vi "Test Passing Method.vi"(8 "error in (no error)":errorcluster, 11 "Test In Library in":refnum<class "Test In Library.lvclass">) -> (0 "error out":errorcluster, 3 "Test In Library out":refnum<class "Test In Library.lvclass">)   [LabVIEW 2020, in "library.lvlib" / "Test In Library.lvclass"]
uses:
  Test In Library.lvclass
  Test In Library.lvclass/Test In Library.ctl
  Core/LUnit Test Case/LUnit Test Case.lvclass
  C:/git/astemes-lunit/source/Core/LUnit Test Case/LUnit Test Case.lvclass
  C:/git/astemes-lunit/source/Core/Runnable/Runnable.lvclass
  C:/git/astemes-lunit/source/Tests/Test Suite Tests/lvlib/Test In Library.lvclass
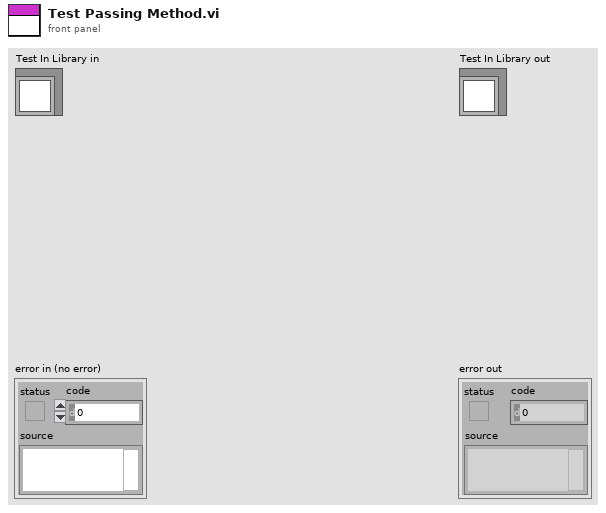
[diagram p1: front panel]
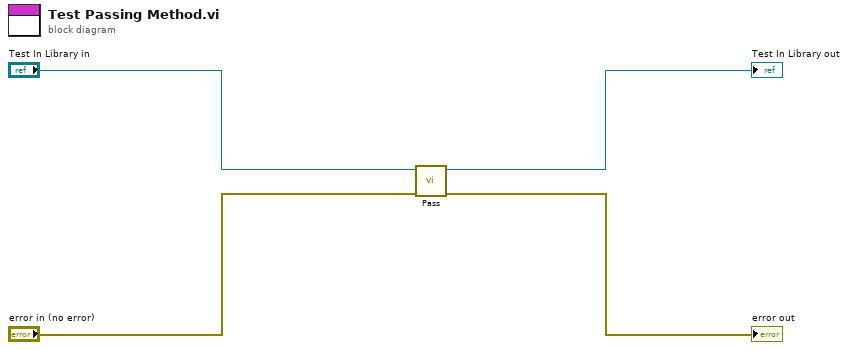
[diagram p0: block diagram]
diagram:
  n1 = call "Pass.vi"("error in (no error)"="error in (no error)", "LUnit Test Case In"="Test In Library in") -> ("error out"=→"error out":errorcluster, "LUnit Test Case Out"=→"Test In Library out":refnum<class "Test In Library.lvclass">)  [unwired: 8 in]
